vi "Create Snapshot Transaction List.vi"(9 "Combined LBCBs":bool, 11 "Number of LBCBs":T1) -> (2 "Transactions":T2[](array[typedef]))   [LabVIEW 2009]
uses:
  Dataset Transaction Id.ctl
  Dataset Source.ctl
  Dataset Type.ctl
  Apps/Yes No Button.ctl
  Data Access Objects/Application/Number Of LBCBs.ctl
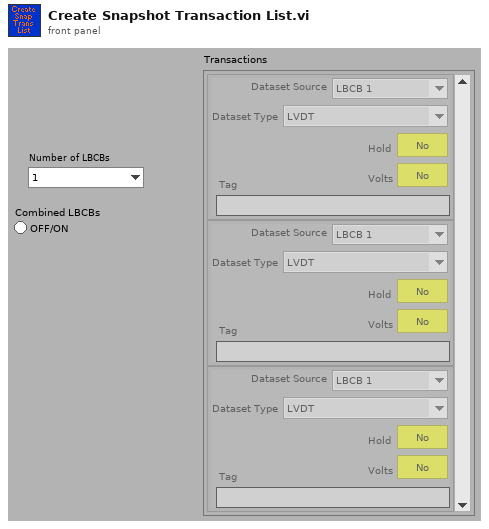
[diagram p1: front panel]
types:
  T1 = typedef "Number Of LBCBs.ctl" = enum16{"1", "2"}
  T2 = typedef "Dataset Transaction Id.ctl" = cluster{"Dataset Source":T3, "Dataset Type":T4, "Hold":T5, "Volts":T5, "Tag":string}
  T3 = typedef "Dataset Source.ctl" = enum16{"LBCB 1", "LBCB 2", "Combined", "External Sensors"}
  T4 = typedef "Dataset Type.ctl" = enum16{"LVDT", "Load Cell", "Actuator Command", "Servo Error", "Displacement Command", "Displacement", "Force"}
  T5 = typedef "Yes No Button.ctl" = bool
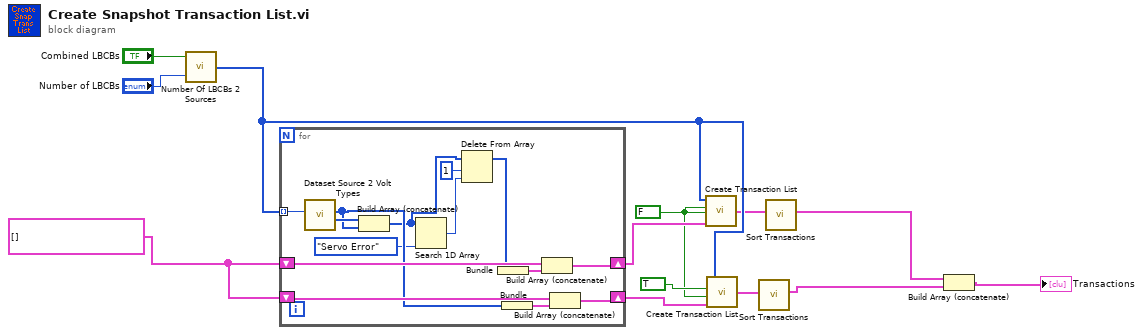
[diagram p0: block diagram]
diagram:
  w1 = T5 FALSE ("Hold")
  w10 = cluster{"Hold Types":T4[]}[] []
  n1 = call "Number Of LBCBs 2 Sources.vi"("Number of LBCBs"="Number of LBCBs", "Combined LBCBs"="Combined LBCBs") -> ("Sources"=w11:T3[])
  n2 = for {
    tunnel: w11 -> [w27] mode=indexing
    shift-right: [w26] -> w9
    shift-left: w10 -> [w25]
    shift-right: [w22] -> w5
    shift-left: w10 -> [w21]
    n3 = call "Dataset Source 2 Volt Types.vi"("Dataset Source"=w27) -> ("No Volt Types Out"=w20:T4[], "Volt Types"=w19:T4[])  [unwired: 9 in]
    n4 = Build Array (concatenate)(w20, w19) -> (w15:T4[])
    n5 = Search 1D Array(1D array=w15, element=Dataset_Type."Servo Error") -> (index of element=w17:i32)  [unwired: 1 in]
    n6 = Delete From Array(array=w15, length=1, index=w17) -> (array with subset deleted=w14:T4[])  [unwired: 1 out]
    n7 = Bundle(w14) -> (w24:cluster{T4[]})  [unwired: 1 in]
    n8 = Bundle("Volt Types"=w19) -> (w23:cluster{"Volt Types":T4[]})  [unwired: 1 in]
    n9 = Build Array (concatenate)(w25, w24) -> (w26:cluster{"Hold Types":T4[]}[])
    n10 = Build Array (concatenate)(w21, w23) -> (w22:cluster{"Volt Types":T4[]}[])
  }
  n11 = call "Create Transaction List.vi"("Source Types"=w9, "Hold"=w1, "Volts"=w1, "Sources"=w11) -> ("Transactions"=w6:T2[])
  n12 = call "Create Transaction List.vi"("Source Types"=w5, "Hold"=w1, "Volts"=TRUE, "Sources"=w11) -> ("Transactions"=w7:T2[])
  n13 = call "Sort Transactions.vi"("Transactions In"=w7) -> ("Transactions Out"=w2:T2[])  [unwired: 10 in]
  n14 = call "Sort Transactions.vi"("Transactions In"=w6) -> ("Transactions Out"=w3:T2[])  [unwired: 10 in]
  n15 = Build Array (concatenate)(w3, w2) -> (→"Transactions":T2[])
